vi "ESNLookup.vi"(6 "ESN":string, 8 "error in":errorcluster) -> (0 "error out":errorcluster, 4 "MSN":string, 5 "success":bool)   [LabVIEW 2018]
uses:
  <vilib>/Utility/file.llb/Read Delimited Spreadsheet (string).vi
panel:
  out "table":string[][](array[string])
  in  "esn/msn table (.csv)":path=path "C:/RageATE/Automated Tests/Tetra WAM/Utilities/ESN_Master_Table.csv"
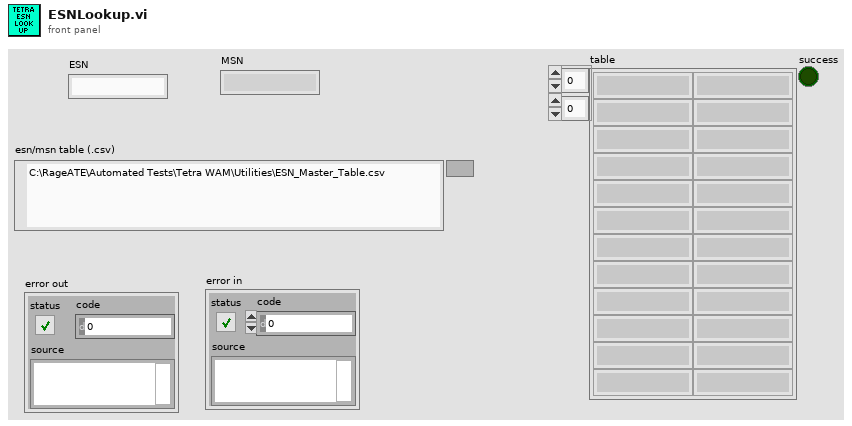
[diagram p1: front panel]
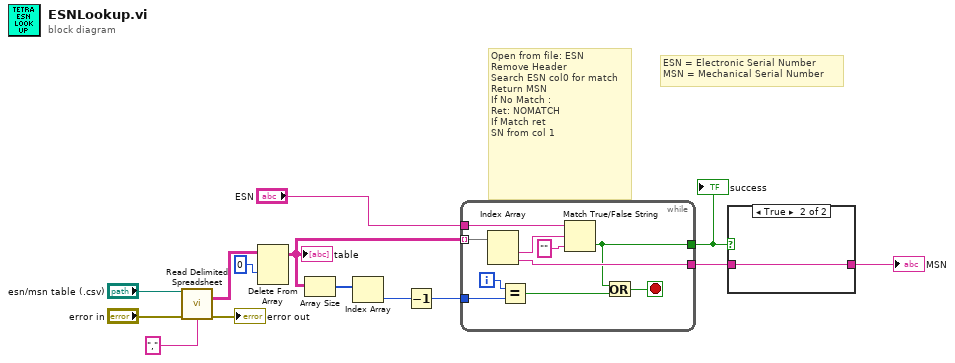
[diagram p0: block diagram]
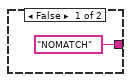
[diagram p2: hidden frame]
diagram:
  # "ESN = Electronic Serial Number\nMSN = Mechanical Serial Number"
  # "Open from file: ESN\nRemove Header\nSearch ESN col0 for match\nReturn MSN\nIf No Match :\nRet: NOMATCH\nIf Match ret\nSN from col 1"
  n1 = call-poly <vilib>:"Read Delimited Spreadsheet.vi"("file path (dialog if empty)"="esn/msn table (.csv)", "error in (no error)"="error in", "delimiter (\\t)"="," ("delimiter (\\t)")) -> ("all rows"=w12:string[][], "error out"=→"error out":errorcluster)  [unwired: 7 in, 4 out]
  n2 = Delete From Array(array=w12, index (row)=0) -> (array with subset deleted=w7:string[][])  [unwired: 2 in, 1 out]
  "table" <- w7
  n3 = Array Size(array=w7) -> (size(s)=w6:i32[])
  n4 = Index Array(array=w6) -> (element=w3:i32)  [unwired: 1 in]
  n5 = Decrement(x=w3) -> (x-1=w1:i32)
  n6 = while {
    tunnel: "ESN" -> [w24]
    tunnel: w7 -> [w23] mode=indexing
    tunnel: [w20] -> w5
    tunnel: w1 -> [w18]
    tunnel: [w15] -> w2
    i -> [w19]
    stop <- w16 stop-if-true
    n7 = Index Array(array=w23) -> (element #1=w22:string, element #2=w20:string)  [unwired: 2 in]
    n8 = Equal?(x=w19, y=w18) -> (x = y?=w17:bool)
    n9 = Match True/False String(2:"" ("false string"), 3:w22, 4:w24) -> (0:w15:bool)  [unwired: 1 out]
    n10 = Or(x=w15, y=w17) -> (x .or. y?=w16:bool)
  }
  "success" <- w2
  n11 = case shown="True" w2 {
    tunnel: w5 -> [_ w26]
    tunnel: ["NOMATCH" ("String") w26] -> w4
    frame False {
    }
    frame True {
    }
  }
  "MSN" <- w4
